vi "Stop Core.vi"(10 "final error code":i32, 11 "Abstract Display in":refnum<class "Abstract Display.lvclass">) -> (3 "Abstract Display out":refnum<class "Abstract Display.lvclass">)   [LabVIEW 2014, in "Display Panel.lvlib" / "Abstract Display.lvclass"]
doc: "(<B>Filename</B>: Actor Framework.lvlib:Actor.lvclass:Stop Core.vi)\n\nDefines what the actor does before it stops. Use the <B>final error code</B> input to determine whether the actor shut down in response to an error.\n\nBy default, this method does nothing. A descendant class may override it to define behavior, such as shutting down any processes the actor initiated in its override of the Actor Core method."
uses:
  Abstract Display.lvclass
  <vilib>/ActorFramework/Message Enqueuer/Message Enqueuer.lvclass/Message Enqueuer.ctl
  <vilib>/ActorFramework/Message Enqueuer/Enqueue.vi
  <vilib>/ActorFramework/Message Priority Queue/Priority Enqueue.vi
  <vilib>/ActorFramework/Stop Msg/Stop Msg.lvclass
  <vilib>/ActorFramework/Actor/Actor.lvclass
panel:
  out "error out":errorcluster
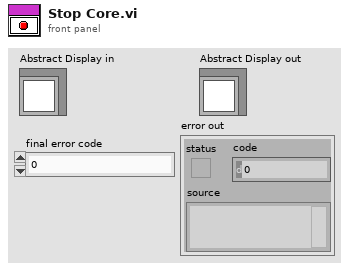
[diagram p1: front panel]
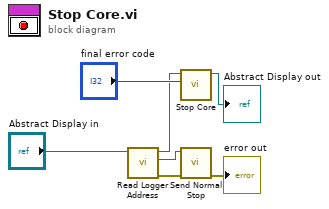
[diagram p0: block diagram]
diagram:
  n1 = call-dynamic "Read Logger Address .vi"("Abstract Display in"="Abstract Display in") -> ("error out"=w2:errorcluster, "Actor Framework:Message Enqueuer"=w3:refnum<class "Message Enqueuer.lvclass">, "Abstract Display out"=w4:refnum<class "Abstract Display.lvclass">)  [unwired: 8 in]
  n2 = call-parent "Stop Core.vi"("final error code"="final error code", "Actor in"=w4) -> ("Actor out"=→"Abstract Display out":refnum<class "Abstract Display.lvclass">)  [unwired: 9 in]
  n3 = call <vilib>:"Send Normal Stop.vi"("error in (no error)"=w2, "Message Enqueuer"=w3) -> ("error out"=→"error out":errorcluster)  [unwired: 9 in]
